vi "make_request.vi"(8 "Error in":errorcluster, 10 "Content-Type":string, 11 "Device In":T1) -> (0 "error out":errorcluster, 1 "error":i32, 2 "Comm":T2, 3 "Device Out":T1)   [LabVIEW 2019]
uses:
  <userlib>/IoT Devices/_subVIs/HTTPComm.ctl
  Cluster.ctl
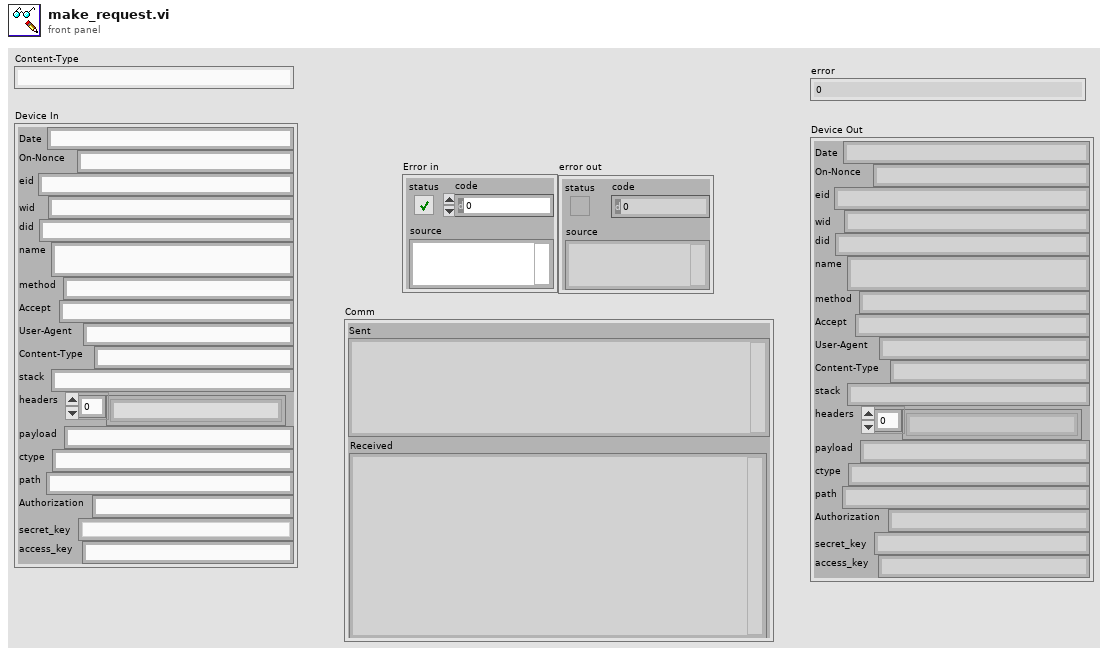
[diagram p1: front panel]
types:
  T1 = typedef "Cluster.ctl" = cluster{"Date":string, "On-Nonce":string, "eid":string, "wid":string, "did":string, "name":string, "method":string, "Accept":string, "User-Agent":string, "Content-Type":string, "stack":string, "headers":string[], "payload":string, "ctype":string, "path":string, "Authorization":string, "secret_key":string, "access_key":string}
  T2 = typedef "HTTPComm.ctl" = cluster{"url":string, "sent headers":string, "sent body":string, "headers":string, "body":string, "Sent":string, "Received":string}
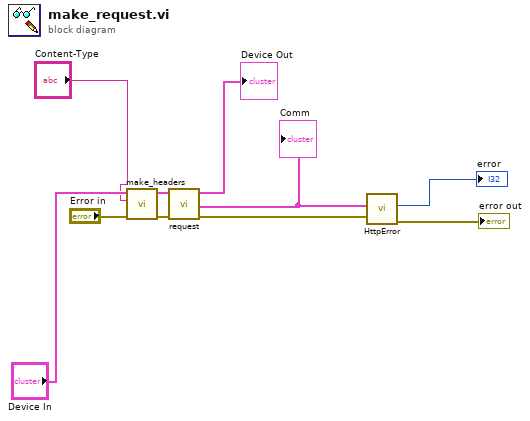
[diagram p0: block diagram]
diagram:
  n1 = call "make_headers.vi"("Error in"="Error in", "Content-Type"="Content-Type", "Device In"="Device In") -> ("Error Out"=w9:errorcluster, "Device Out"=w10:T1)  [unwired: 7 in]
  n2 = call "request.vi"("Device In"=w10, "error in"=w9) -> ("Device Out"=→"Device Out":T1, "Comm"=w4:T2, "error out"=w3:errorcluster)  [unwired: 6 in]
  "Comm" <- w4
  n3 = call "HttpError.vi"("error in (no error)"=w3, "Comm"=w4) -> ("error out"=→"error out":errorcluster, "error"=→"error":i32)  [unwired: 8 in]
